vi "All Set Value.vi"(8 "error in (no error)":errorcluster, 10 "Value (F)":bool, 11 "MCListbox with Checkboxes in":refnum<class "MCListbox with Checkboxes.lvclass">) -> (0 "error out":errorcluster, 3 "MCListbox with Checkboxes out":refnum<class "MCListbox with Checkboxes.lvclass">)   [LabVIEW 2016, in "MCListbox with Checkboxes.lvclass"]
uses:
  MCListbox with Checkboxes.lvclass
  MCListbox with Checkboxes.lvclass/MCListbox with Checkboxes.ctl
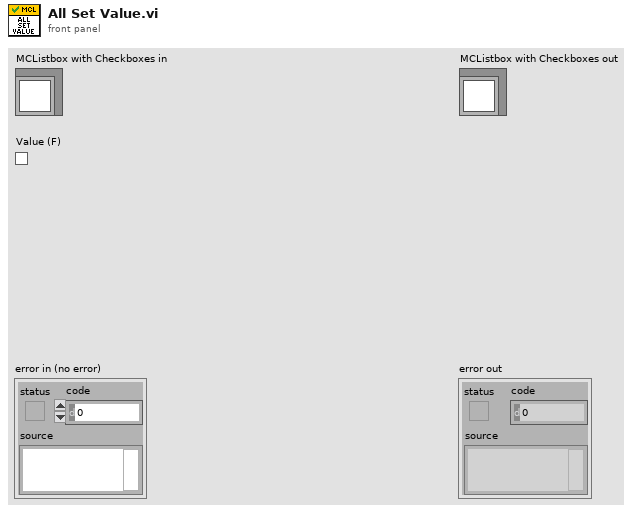
[diagram p1: front panel]
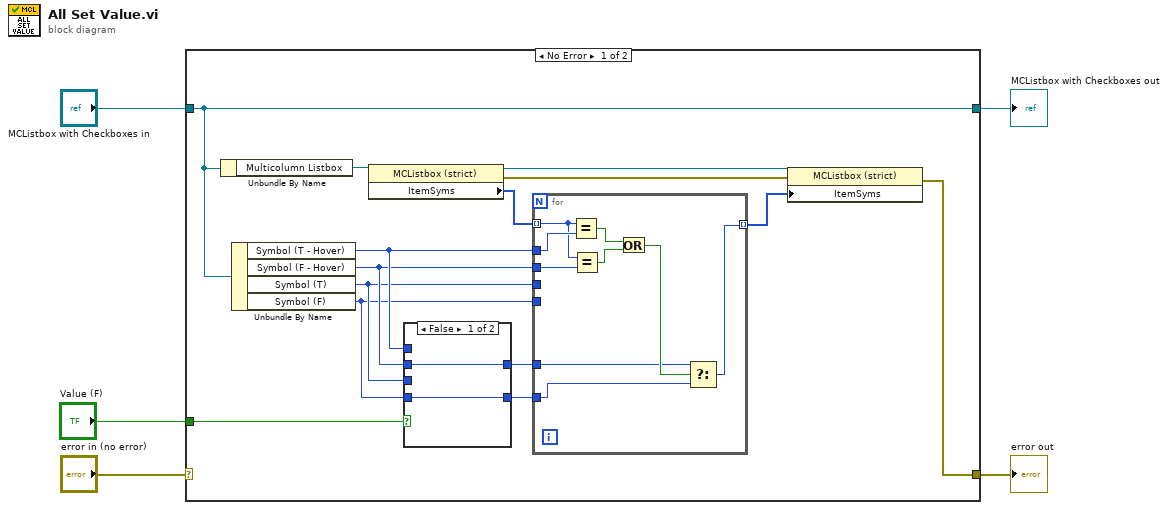
[diagram p0: block diagram]
diagram:
  n1 = case shown="No Error" "error in (no error)" {
    selector: "error in (no error)" -> [_ w34]
    tunnel: [w6 w34] -> w4
    tunnel: [w17 w33] -> w2
    tunnel: "MCListbox with Checkboxes in" -> [w17 w33]
    tunnel: "Value (F)" -> [w16 _]
    frame No Error {
      n2 = Unbundle By Name(w17) -> ("Multicolumn Listbox"=w19:refnum<vi>)
      n3 = Unbundle By Name(w17) -> ("Symbol (T - Hover)"=w15:i32, "Symbol (F - Hover)"=w14:i32, "Symbol (T)"=w13:i32, "Symbol (F)"=w12:i32)
      n4 = property class="MCListbox (strict)"(reference=w19) -> (reference out=w9:refnum<vi>, error out=w8:errorcluster, "ItemSyms"=w18:i32[])  [unwired: 1 in]
      n5 = case shown="False" w16 {
        tunnel: w15 -> [_ w23]
        tunnel: w14 -> [w21 _]
        tunnel: w13 -> [_ w22]
        tunnel: w12 -> [w20 _]
        tunnel: [w21 w23] -> w11
        tunnel: [w20 w22] -> w10
        frame False {
        }
        frame True {
        }
      }
      n6 = for {
        tunnel: w18 -> [w30] mode=indexing
        tunnel: w15 -> [w32]
        tunnel: w14 -> [w31]
        tunnel: w13 -> [_]
        tunnel: w12 -> [_]
        tunnel: w11 -> [w26]
        tunnel: w10 -> [w25]
        tunnel: [w24] -> w7 mode=indexing
        n7 = Equal?(x=w30, y=w32) -> (x = y?=w29:bool)
        n8 = Equal?(x=w30, y=w31) -> (x = y?=w28:bool)
        n9 = Or(x=w29, y=w28) -> (x .or. y?=w27:bool)
        n10 = Select(t=w26, s=w27, f=w25) -> (s? t:f=w24:i32)
      }
      n11 = property class="MCListbox (strict)"(reference=w9, error in=w8, "ItemSyms"=w7) -> (error out=w6:errorcluster)  [unwired: 1 out]
    }
    frame Error {
    }
  }
  "error out" <- w4
  "MCListbox with Checkboxes out" <- w2
